vi "Read Haskel.vi"(0 "FPGA API in":refnum<class "FPGA API Mock.lvclass">, 11 "error in (no error)":errorcluster) -> (4 "FPGA API out":refnum<class "FPGA API Mock.lvclass">, 6 "Haskel AO Value":dbl, 15 "error out":errorcluster)   [LabVIEW 2019, in "FPGA API Mock.lvclass"]
uses:
  FPGA API Mock.lvclass
  FPGA API Mock.lvclass/FPGA API Mock.ctl
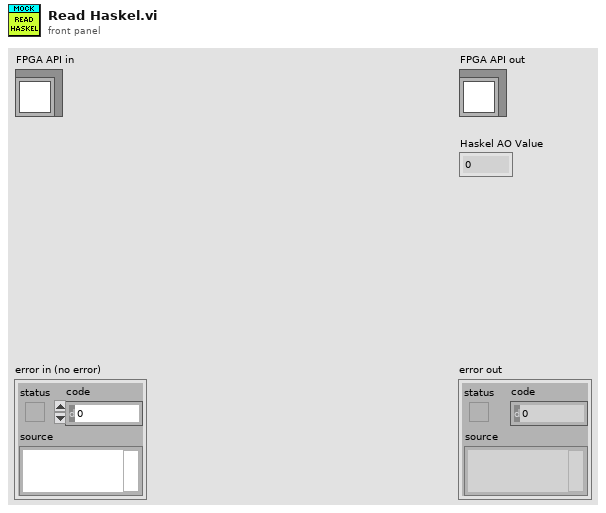
[diagram p1: front panel]
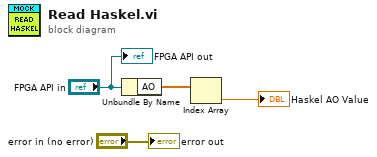
[diagram p0: block diagram]
diagram:
  n1 = Unbundle By Name("FPGA API in") -> ("AO"=w2:dbl[])
  n2 = Index Array(array=w2) -> (element=→"Haskel AO Value":dbl)  [unwired: 1 in]
  "error out" <- "error in (no error)"
  "FPGA API out" <- "FPGA API in"
